vi "Compute Single Buffer Length.vi"(2 "Duration (ms)":dbl, 3 "Sampling rate (Hz)":dbl) -> (0 "Double buffer length":i32, 1 "Sampling rate (out)":dbl)   [LabVIEW 2015]
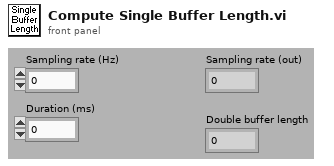
[diagram p1: front panel]
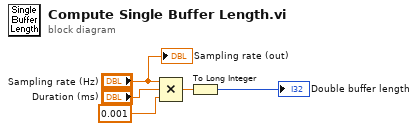
[diagram p0: block diagram]
diagram:
  n1 = Compound Arithmetic op=MULTIPLY("Sampling rate (Hz)", "Duration (ms)", 0.001) -> (w5:dbl)
  n2 = To Long Integer(number=w5) -> (32bit integer=→"Double buffer length":i32)
  "Sampling rate (out)" <- "Sampling rate (Hz)"
